vi "Get_Current_Scan_client.vi"(0 "ADAM Ch Names":string[](array[string])=["EnFlo Tun:Ultrasonic:Fixed"]) -> (1 "Ch Description Array":T1[](array[typedef]) {"Duty" format="%016b"; "D" format="%#_5g"; "C" format="%#_5g"; "B" format="%#_5g"; "A" format="%#_5g"}, 2 "String values":string[](array[string]), 3 "Numerical Values":dbl[](array[numeric]) format="%.9f")   [LabVIEW 2017]
uses:
  Sub VIs/ADAM Controls/Ch_description_ADAM.ctl
  Sub VIs/ADAM Controls/Module_type_ADAM.ctl
  Sub VIs/ADAM Controls/Function_ADAM.ctl
  Sub VIs/ADAM Controls/Channel_State.ctl
  Sub VIs/ADAM Controls/Calib_type_ADAM.ctl
  Sub VIs/ADAM Controls/Address.ctl
  Anemometry/Anemometry Sub Vis/Controls/Global_mode.ctl
  Anemometry/Anemometry Sub Vis/Globals/Preference_global.vi
panel:
  in  "server type":refnum<vi>
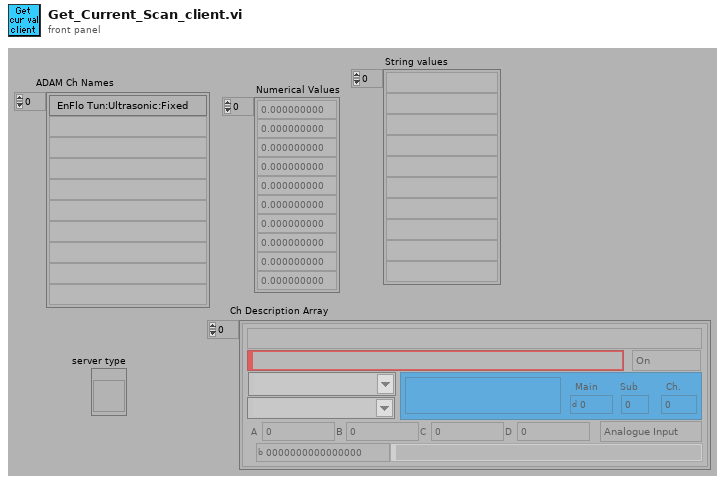
[diagram p1: front panel]
types:
  T1 = typedef "Ch_description_ADAM.ctl" = cluster{"Ch Name":string, "Type":T2, "Function":T3, "Ch State":T4, "Calibration type":T5, "A":dbl, "B":dbl, "C":dbl, "D":dbl, "Comments":string, "Address":T6, "String":string, "Duty":u16}
  T2 = typedef "Module_type_ADAM.ctl" = string
  T3 = typedef "Function_ADAM.ctl" = enum16{"Analogue Input", "Digital Input", "Event counter", "Event rate", "Analogue Output", "Digital Output", "Relay Output"}
  T4 = typedef "Channel_State.ctl" = enum16{"On", "Off", "Always On", "Always Off"}
  T5 = typedef "Calib_type_ADAM.ctl" = string
  T6 = typedef "Address.ctl" = cluster{"Main":i32, "Ch.":i32, "Sub":i32, "Port Name":string}
  T7 = typedef "Server_Comms.ctl" = enum16{"Server Link Healthy", "Do Not Link To Server"}
  T8 = typedef "Global_mode.ctl" = enum16{"Read Global", "Load Global From File", "Write Global to File"}
  T9 = typedef "Update_scan_value.ctl" = cluster{"Channel Name":string, "New Value":dbl}
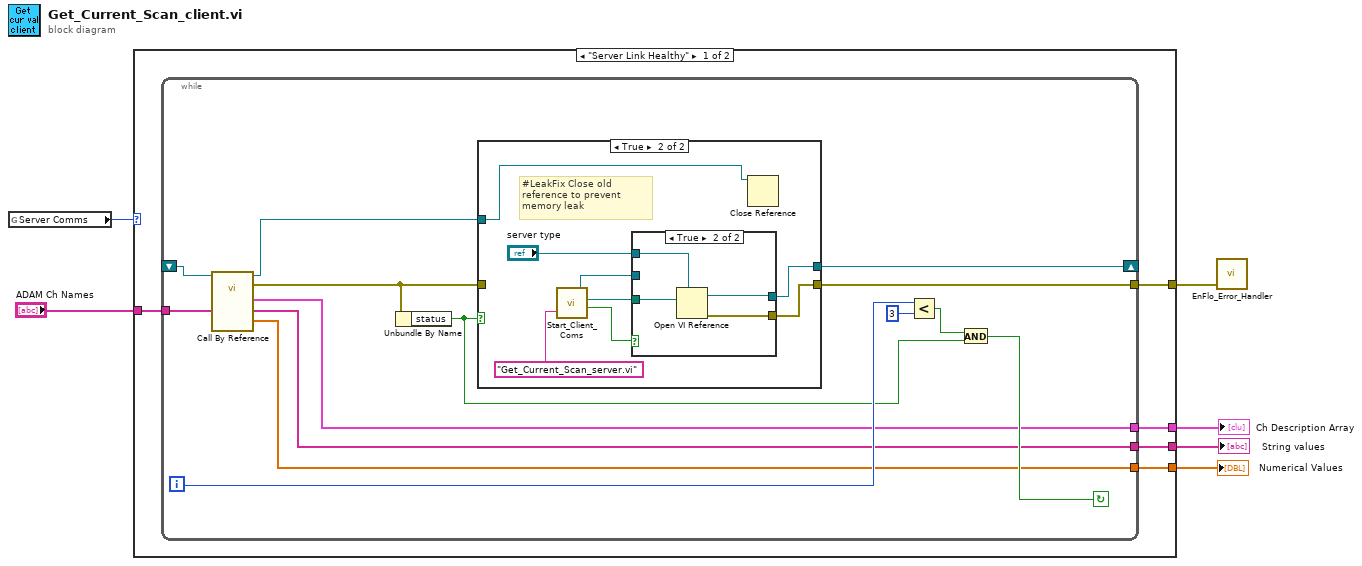
[diagram p0: block diagram]
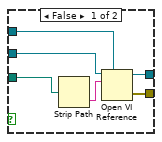
[diagram p3: hidden frame]
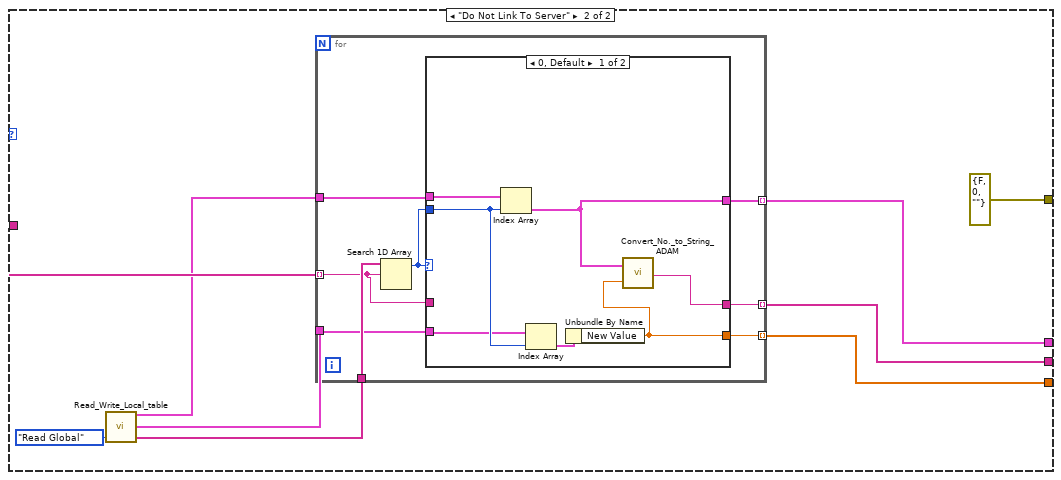
[diagram p4: hidden frame]
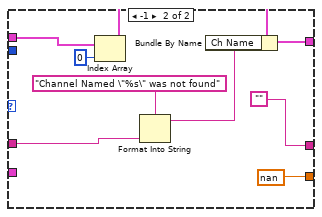
[diagram p5: hidden frame]
diagram:
  n1 = global read "Preference_global.vi" "Server Comms"() -> (w6:T7)
  n2 = case shown="\"Server Link Healthy\"" w6 {
    tunnel: [w11 errorcluster {"status"=FALSE, "code"=0, "source"=""}] -> w5
    tunnel: "ADAM Ch Names" -> [w10 w51]
    tunnel: [w7 w46] -> w1
    tunnel: [w9 w49] -> w3
    tunnel: [w8 w48] -> w2
    frame "Server Link Healthy" {
      n3 = while {
        tunnel: [w16] -> w8
        tunnel: [w17] -> w9
        tunnel: w10 -> [w23]
        tunnel: [w18] -> w11
        shift-left: _ -> [w25]
        shift-right: [w20] -> _
        tunnel: [w15] -> w7
        i -> [w19]
        stop <- w24 continue-if-true
        n4 = call-by-ref "Call By Reference"(reference=w25, "Desired Channels"=w23) -> (reference out=w22:refnum<vi>, error out=w21:errorcluster, "Ch Description Array"=w15:T1[], "String values"=w17:string[], "Numerical Values"=w16:dbl[])  [unwired: 1 in]
        n5 = Unbundle By Name(w21) -> ("status"=w14:bool)
        n6 = case shown="True" w14 {
          tunnel: [w26 w31] -> w20
          tunnel: [w27 w29] -> w18
          tunnel: w21 -> [w27 _]
          tunnel: w22 -> [w26 w28]
          frame False {
          }
          frame True {
            # "#LeakFix Close old reference to prevent memory leak"
            n7 = call "Start_Client_Coms.vi"("VI name to run on server"="Get_Current_Scan_server.vi") -> ("LabVIEW application reference"=w33:refnum<vi>, "Checked VI name"=w34:path, "Local Call"=w32:bool)  [unwired: 1 in, 1 out]
            n8 = case shown="True" w32 {
              tunnel: [w39 w45] -> w31
              tunnel: "server type" -> [w38 w44]
              tunnel: w34 -> [w37 w43]
              tunnel: w33 -> [w36 _]
              tunnel: [w40 w42] -> w29
              frame False {
                n9 = Strip Path(path=w37) -> (name=w41:string)  [unwired: 1 out]
                n10 = Open VI Reference(type specifier VI Refnum (for type only)=w38, application reference (local)=w36, vi path=w41) -> (vi reference=w39:refnum<vi>, error out=w40:errorcluster)  [unwired: 1 in, 2 out]
              }
              frame True {
                n11 = Open VI Reference(type specifier VI Refnum (for type only)=w44, vi path=w43) -> (vi reference=w45:refnum<vi>, error out=w42:errorcluster)  [unwired: 1 in, 3 out]
              }
            }
            n12 = Close Reference(reference=w28) -> ()  [unwired: 1 in, 1 out]
          }
        }
        n13 = Less?(x=w19, y=3) -> (x < y?=w13:bool)
        n14 = And(x=w13, y=w14) -> (x .and. y?=w24:bool)
      }
    }
    frame "Do Not Link To Server" {
      n15 = call "Read_Write_Local_table.vi"("Mode"=Global_mode."Read Global") -> ("Ch Names"=w52:string[], "Ch Values Out"=w47:T9[], "Channels Descriptions Out"=w50:T1[])  [unwired: 2 in]
      n16 = for {
        tunnel: w52 -> [w62]
        tunnel: w51 -> [w55] mode=indexing
        tunnel: w50 -> [w60]
        tunnel: [w59] -> w46 mode=indexing
        tunnel: [w58] -> w49 mode=indexing
        tunnel: [w57] -> w48 mode=indexing
        tunnel: w47 -> [w56]
        n17 = Search 1D Array(1D array=w62, element=w55) -> (index of element=w61:i32)  [unwired: 1 out]
        n18 = case shown="0, Default" w61 {
          tunnel: w61 -> [w68 _]
          tunnel: w60 -> [w69 w77]
          tunnel: [w65 w75] -> w59
          tunnel: [w63 ""] -> w58
          tunnel: [w64 nan] -> w57
          tunnel: w56 -> [w67 _]
          tunnel: w55 -> [_ w72]
          frame 0, Default {
            n19 = Index Array(array=w69, index=w68) -> (element=w65:T1)
            n20 = Index Array(array=w67, index=w68) -> (element=w66:T9)
            n21 = Unbundle By Name(w66) -> ("New Value"=w64:dbl)
            n22 = call "Convert_No._to_String_ADAM.vi"("Input number"=w64, "Ch Description"=w65) -> ("Output sting"=w63:string)
          }
          frame -1 {
            n23 = Index Array(array=w77, index=0 ("Index")) -> (element=w76:T1)
            n24 = Format Into String(format string="Channel Named \"%s\" was not found" ("Format String"), w72) -> (resulting string=w70:string)  [unwired: 2 in, 1 out]
            n25 = Bundle By Name(cluster=w76, "Ch Name"=w70) -> (w75:T1)
          }
        }
      }
    }
  }
  "Ch Description Array" <- w1
  "String values" <- w3
  "Numerical Values" <- w2
  n26 = call "EnFlo_Error_Handler.vi"("error in (no error)"=w5) -> ()  [unwired: 2 in, 3 out]
